vi "Connect Valid Terminals.vi"(8 "error in (no error)":errorcluster, 10 "Sink Term":refnum<vi>, 11 "Source Term":refnum<vi>) -> (0 "error out":errorcluster, 3 "Connection Made?":bool)   [LabVIEW 2016]
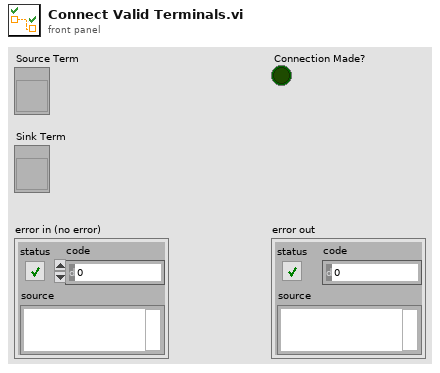
[diagram p1: front panel]
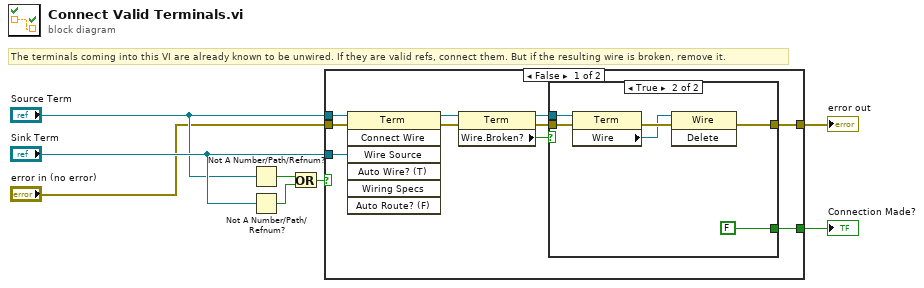
[diagram p0: block diagram]
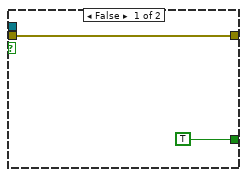
[diagram p2: hidden frame]
diagram:
  # "The terminals coming into this VI are already known to be unwired. If they are valid refs, connect them. But if the resulting wire is broken, remove it."
  n1 = Not A Number/Path/Refnum?(number/path/refnum="Source Term") -> (NaN/Path/Refnum?=w5:bool)
  n2 = Not A Number/Path/Refnum?(number/path/refnum="Sink Term") -> (NaN/Path/Refnum?=w6:bool)
  n3 = Or(x=w5, y=w6) -> (x .or. y?=w7:bool)
  n4 = case shown="False" w7 {
    tunnel: [w10 w27] -> w2
    tunnel: [w9 _] -> w3
    tunnel: "error in (no error)" -> [w18 w27]
    tunnel: "Source Term" -> [w17 _]
    tunnel: "Sink Term" -> [w16 _]
    frame False {
      n5 = invoke class="Term" method="Connect Wire"(reference=w17, error in=w18, "Wire Source"=w16) -> (reference out=w14:refnum<vi>, error out=w15:errorcluster)  [unwired: 4 in, 5 out]
      n6 = property class="Term"(reference=w14, error in=w15) -> (reference out=w11:refnum<vi>, error out=w13:errorcluster, "Wire.Broken?"=w12:bool)
      n7 = case shown="True" w12 {
        tunnel: w13 -> [w20 w24]
        tunnel: w11 -> [_ w25]
        tunnel: [w20 w21] -> w10
        tunnel: [TRUE FALSE] -> w9
        frame False {
        }
        frame True {
          n8 = property class="Term"(reference=w25, error in=w24) -> (error out=w23:errorcluster, "Wire"=w22:refnum<vi>)  [unwired: 1 out]
          n9 = invoke class="Wire" method="Delete"(reference=w22, error in=w23) -> (error out=w21:errorcluster)  [unwired: 1 in, 2 out]
        }
      }
    }
    frame True {
    }
  }
  "Connection Made?" <- w3
  "error out" <- w2
